vi "Start.vi"(8 "error in (no error)":errorcluster, 11 "Debug View In":refnum<class "Debug View.lvclass">) -> (0 "error out":errorcluster, 3 "Debug View Out":refnum<class "Debug View.lvclass">)   [LabVIEW 2020, in "Debug View.lvclass"]
doc: "This VI starts the process which runs asyncronously. The VI blocks the execution until the process has reached its' running state, or the specified timeout expires."
uses:
  Debug View.lvclass
  Debug View.lvclass/Debug View.ctl
  Private/View Holder.vi
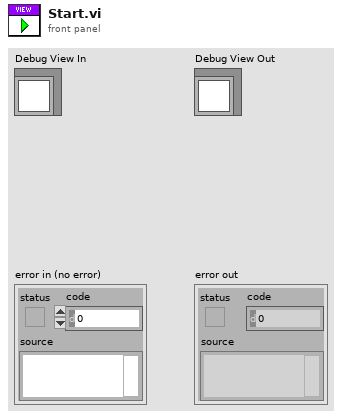
[diagram p1: front panel]
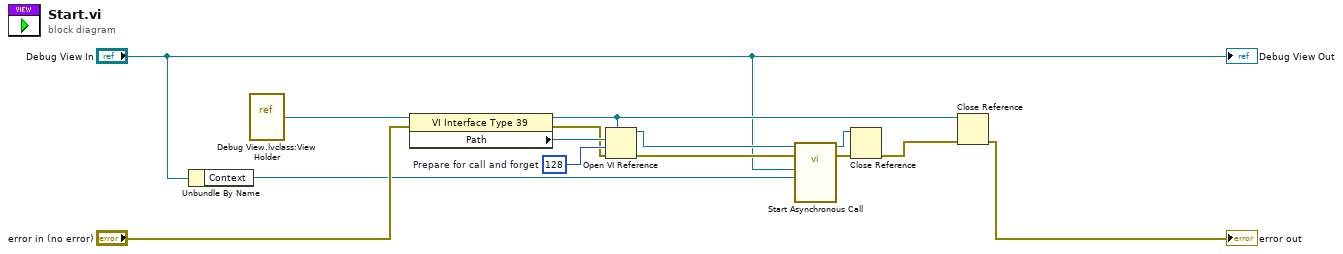
[diagram p0: block diagram]
diagram:
  w13 = 128  # Prepare for call and forget
  n1 = Unbundle By Name("Debug View In") -> ("Context"=w1:refnum<class "Debug Process.lvclass">)
  n2 = vi-ref "Debug View.lvclass:View Holder.vi"() -> (w8:refnum<vi>)
  n3 = property class="VI Interface Type 39"(reference=w8, error in="error in (no error)") -> (reference out=w10:refnum<vi>, error out=w11:errorcluster, "Path"=w12:path)
  n4 = Open VI Reference(type specifier VI Refnum (for type only)=w10, vi path=w12, options=w13, error in (no error)=w11) -> (vi reference=w7:refnum<vi>, error out=w6:errorcluster)  [unwired: 2 in]
  n5 = call-by-ref "Start Asynchronous Call"(reference=w7, error in=w6, "Context"=w1, "Debug View in"="Debug View In") -> (reference out=w3:refnum<vi>, error out=w5:errorcluster)  [unwired: 9 in, 1 out]
  n6 = Close Reference(reference=w3, error in (no error)=w5) -> (error out=w4:errorcluster)
  n7 = Close Reference(reference=w10, error in (no error)=w4) -> (error out=→"error out":errorcluster)
  "Debug View Out" <- "Debug View In"
